vi "VG_YESNON.vi"() -> ()   [LabVIEW 2020]
panel:
  out "OUI/NON":bool
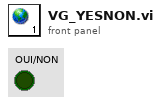
[diagram p1: front panel]
diagram:
